vi "SetZeroPosition.vi"(0 "CmdLib In":refnum<k24>, 5 "DeviceKey In":string, 7 "Device Address In":i32, 9 "Motor":i32, 11 "error in (no error)":errorcluster) -> (4 "CmdLib Out":refnum<k24>, 6 "DeviceKey Out":string, 8 "Device Address Out":i32, 15 "error out":errorcluster)   [LabVIEW 2018]
uses:
  CmdLib.dll
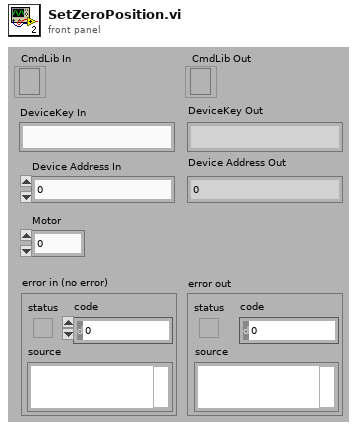
[diagram p1: front panel]
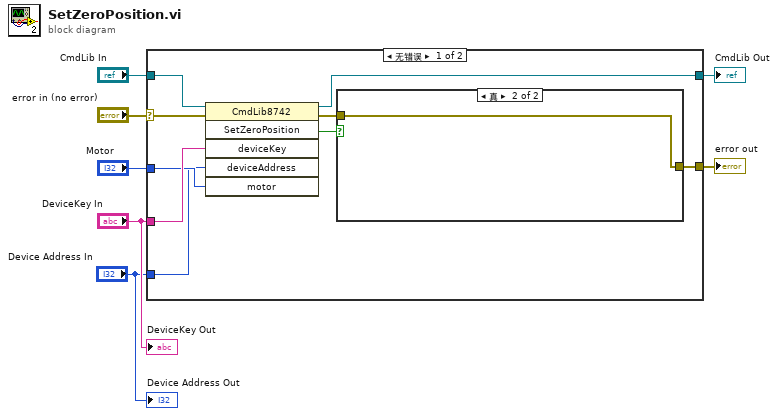
[diagram p0: block diagram]
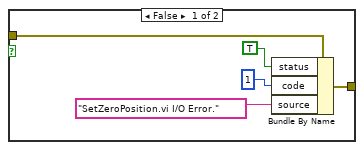
[diagram p2: hidden frame]
diagram:
  n1 = case shown="无错误" "error in (no error)" {
    selector: "error in (no error)" -> [w13 w23]
    tunnel: "CmdLib In" -> [w16 w24]
    tunnel: [w15 w24] -> w6
    tunnel: "Motor" -> [w9 _]
    tunnel: "DeviceKey In" -> [w14 _]
    tunnel: [w10 w23] -> w3
    tunnel: "Device Address In" -> [w8 _]
    frame No Error {
      n2 = invoke class="CmdLib8742" method="SetZeroPosition"(reference=w16, error in=w13, "deviceKey"=w14, "deviceAddress"=w8, "motor"=w9) -> (reference out=w15:refnum<k24>, error out=w11:errorcluster, "SetZeroPosition"=w12:bool)  [unwired: 1 in, 3 out]
      n3 = case shown="真" w12 {
        tunnel: w11 -> [w21 w22]
        tunnel: [w20 w22] -> w10
        frame False {
          n4 = Bundle By Name(cluster=w21, "status"=TRUE, "code"=1, "source"="SetZeroPosition.vi I/O Error.") -> (w20:errorcluster)
        }
        frame True {
        }
      }
    }
    frame Error {
    }
  }
  "error out" <- w3
  "CmdLib Out" <- w6
  "DeviceKey Out" <- "DeviceKey In"
  "Device Address Out" <- "Device Address In"
